vi "Construct_Remaining_Subtrack_101_2_Subtracks-1.vi"(0 "[IN] Still connected\ntracks in group":T2, 1 "[IN] Indexes for Jumps":i32[](array[numeric]), 5 "[IN] Clusters for Re\nconstructed Tracks":T1, 7 "[IN] Index of recon\nstructed tracks":i32, 11 "error IN":errorcluster, 12 "[IN] # column of re\nmaining elongation":i32, 13 "[IN] Indicies of Po\nints Inside Trks":i32[](array[numeric]), 14 "[IN] Indicies of all \nAffected Tracks \n(initial point = 0)":i32[](array[numeric])) -> (6 "[OUT] Clusters for Re\nconstructed Tracks":T1, 15 "error OUT":errorcluster)   [LabVIEW 2013]
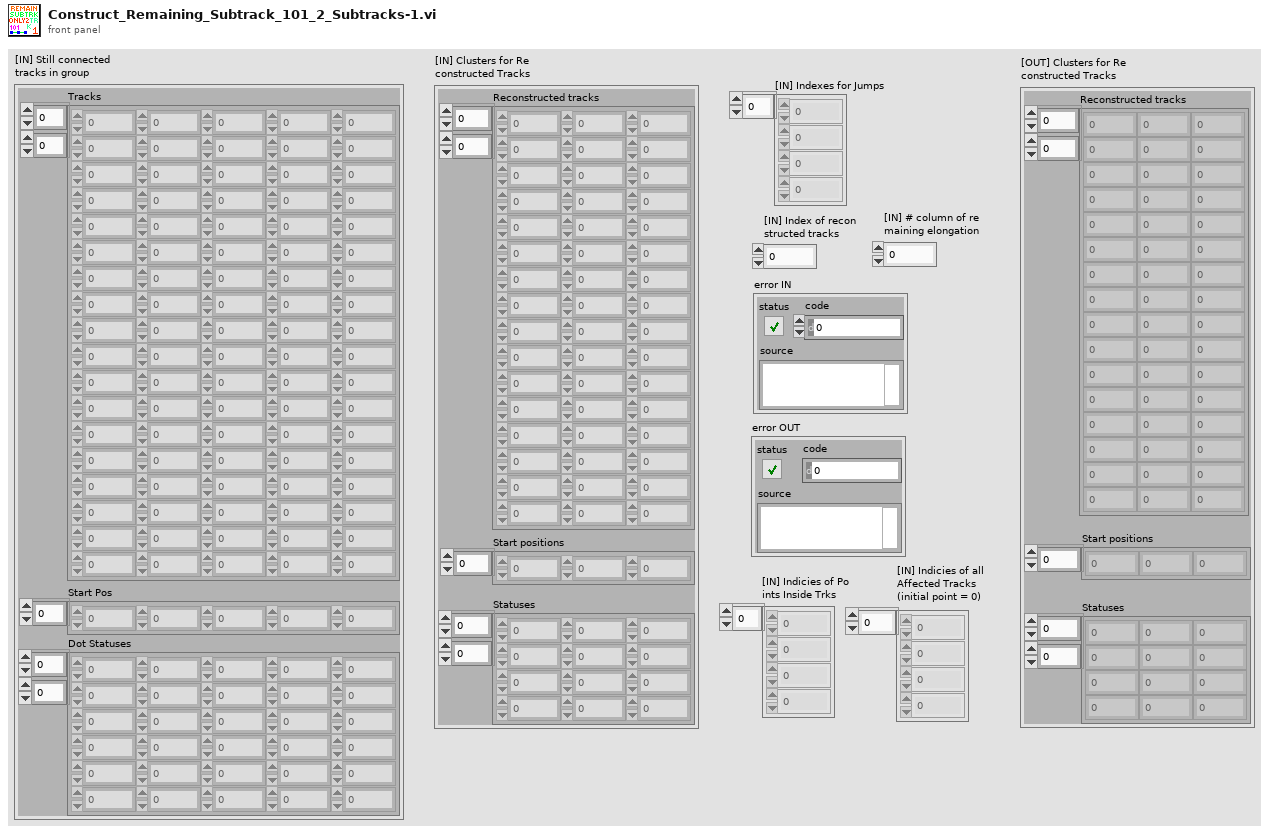
[diagram p1: front panel]
types:
  T1 = cluster{"Reconstructed tracks":dbl[][], "Start positions":i32[], "Statuses":i16[][]}
  T2 = cluster{"Tracks":dbl[][], "Start Pos":i32[], "Dot Statuses":i16[][]}
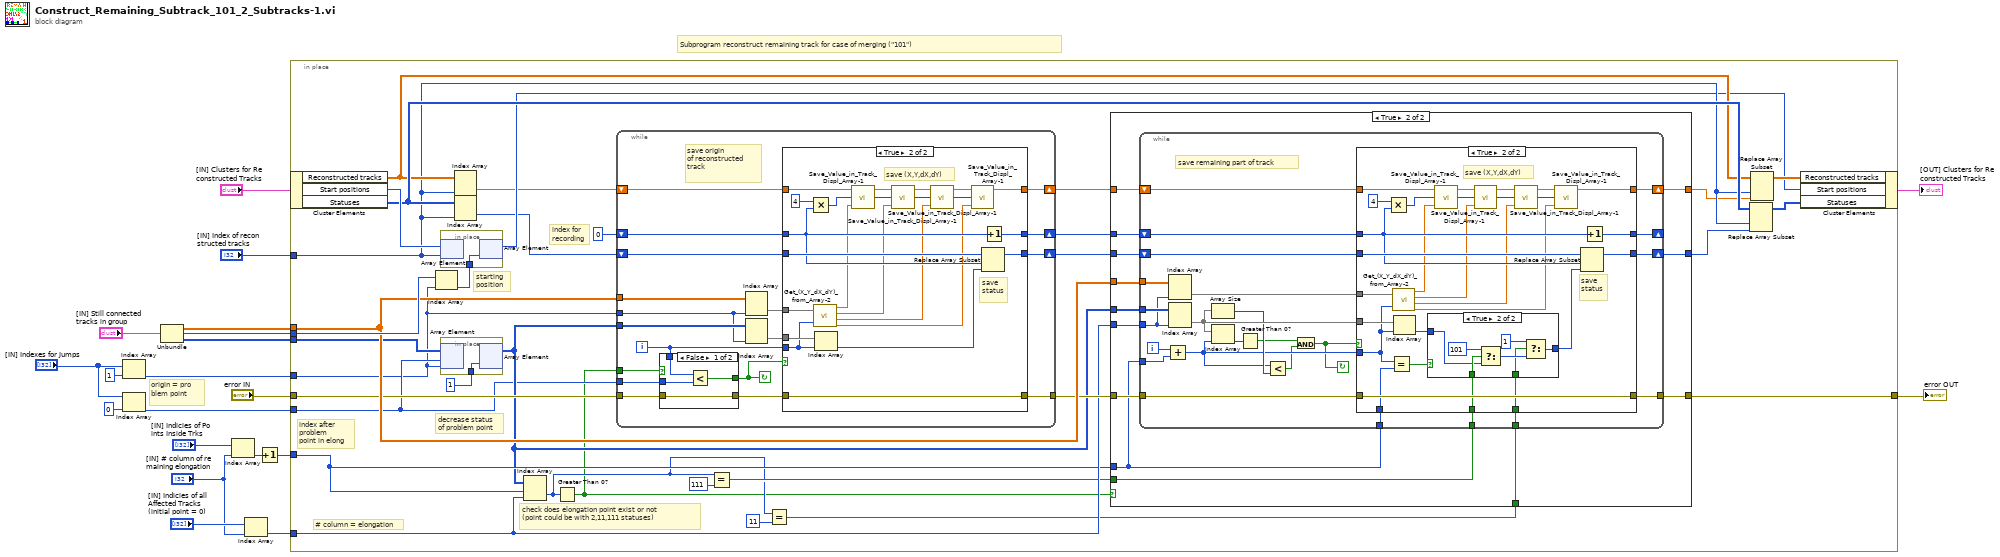
[diagram p0: block diagram]
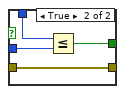
[diagram p5: hidden frame]
diagram:
  # "origin = pro\nblem point"
  # "Subprogram reconstruct remaining track for case of merging (\"101\")"
  n1 = Index Array(array="[IN] Indexes for Jumps", index=1) -> (element=w14:i32)
  n2 = Index Array(array="[IN] Indexes for Jumps", index=0) -> (element=w10:i32)
  n3 = Unbundle("[IN] Still connected\ntracks in group") -> ("Tracks"=w11:dbl[][], "Start Pos"=w12:i32[], "Dot Statuses"=w13:i16[][])
  n4 = Index Array(array="[IN] Indicies of Po\nints Inside Trks", index="[IN] # column of re\nmaining elongation") -> (element=w3:i32)
  n5 = Index Array(array="[IN] Indicies of all \nAffected Tracks \n(initial point = 0)", index="[IN] # column of re\nmaining elongation") -> (element=w5:i32)
  n6 = Increment(x=w3) -> (x+1=w2:i32)
  n7 = in-place {
    in-place-border: "[IN] Index of recon\nstructed tracks" -> [w49]
    in-place-border: w14 -> [w22]
    in-place-border: w13 -> [w29]
    in-place-border: w12 -> [w54]
    in-place-border: w11 -> [w53]
    in-place-border: w10 -> [w27]
    in-place-border: "error IN" -> [w48]
    in-place-border: w5 -> [w33]
    in-place-border: [w44] -> w7
    in-place-border: w2 -> [w32]
    # "decrease status\nof problem point"
    # "check does elongation point exist or not  \n(point could be with 2,11,111 statuses)"
    # "# column = elongation"
    # "index after\nproblem \npoint in elong"
    # "index for\nrecording"
    # "starting\nposition"
    n8 = in-place-cluster #1("[IN] Clusters for Re\nconstructed Tracks") -> ("Reconstructed tracks"=w50:dbl[][], "Start positions"=w52:i32[], "Statuses"=w51:i16[][])
    n9 = Index Array(array=w54, index=w22) -> (element=w43:i32)
    n10 = in-place {
      in-place-border: w43 -> [w189]
      n11 = in-place-array #2(w52, w49) -> ()  [unwired: 1 out]
      n12 = in-place-array #2(w189) -> (w46:i32[])  [unwired: 1 out]
    }
    n13 = in-place {
      in-place-border: i16 1 ("element") -> [w55]
      n14 = in-place-array #3(w29, w27, w22) -> ()  [unwired: 1 out]
      n15 = in-place-array #3(w55) -> (w28:i16[][])  [unwired: 2 out]
    }
    n16 = Index Array(array=w50, index (col)=w49) -> (element=w41:dbl[])  [unwired: 1 in]
    n17 = Index Array(array=w51, index (col)=w49) -> (element=w40:i16[])  [unwired: 1 in]
    n18 = Index Array(array=w28, index (row)=w32, index (col)=w33) -> (element=w24:i16)
    n19 = Greater Than 0?(x=w24) -> (x > 0?=w21:bool)
    n20 = while {
      tunnel: w27 -> [w139]
      tunnel: w53 -> [w153]
      tunnel: w28 -> [w152]
      tunnel: w22 -> [w151]
      shift-right: [w145] -> w39
      shift-left: w41 -> [w150]
      shift-right: [w143] -> w37
      shift-left: w40 -> [w147]
      shift-right: [w144] -> w38
      shift-left: 0 -> [w146]
      tunnel: w48 -> [w137]
      tunnel: [w142] -> w36
      tunnel: w21 -> [w141]
      i -> [w140]
      stop <- w138 continue-if-true
      # "save origin \nof reconstructed \ntrack"
      n21 = case shown="False" w141 {
        tunnel: w140 -> [w157 w161]
        tunnel: w139 -> [w156 w160]
        tunnel: [w155 w159] -> w138
        tunnel: w137 -> [w154 w158]
        tunnel: [w154 w158] -> w136
        frame False {
          n22 = Less?(x=w157, y=w156) -> (x < y?=w155:bool)
        }
        frame True {
          n23 = Less Or Equal?(x=w161, y=w160) -> (x <= y?=w159:bool)
        }
      }
      n24 = Index Array(array=w153, index (col)=w151) -> (element=w149:dbl[])  [unwired: 1 in]
      n25 = Index Array(array=w152, index (col)=w151) -> (element=w148:i16[])  [unwired: 1 in]
      n26 = case shown="True" w138 {
        tunnel: w150 -> [w165 w178]
        tunnel: w149 -> [_ w188]
        tunnel: w148 -> [_ w187]
        tunnel: w140 -> [_ w183]
        tunnel: w147 -> [w163 w185]
        tunnel: [w163 w182] -> w143
        tunnel: [w165 w167] -> w145
        tunnel: w146 -> [w164 w181]
        tunnel: [w164 w180] -> w144
        tunnel: w136 -> [w162 w179]
        tunnel: [w162 w179] -> w142
        frame False {
        }
        frame True {
          # "save (X,Y,dX,dY)"
          # "save\nstatus"
          n27 = Multiply(x=4, y=w181) -> (x*y=w176:i32)
          n28 = call "Get_(X_Y_dX_dY)_from_Array-2.vi"("(X,Y,dX,dY)"=w188, "Index of Displacement"=w183) -> ("X"=w177:dbl, "Y"=w173:dbl, "dX"=w171:dbl, "dY"=w168:dbl)
          n29 = Index Array(array=w187, index=w183) -> (element=w184:i16)
          n30 = call "Save_Value_in_Track_Displ_Array-1.vi"("[IN] Value"=w177, "[IN] Index"=w176, "[IN] Empty tracks\nfor points saving"=w178) -> ("[OUT] Index ++"=w174:i32, "[OUT Track with saved value"=w175:dbl[])  [unwired: 1 in]
          n31 = call "Save_Value_in_Track_Displ_Array-1.vi"("[IN] Value"=w173, "[IN] Index"=w174, "[IN] Empty tracks\nfor points saving"=w175) -> ("[OUT] Index ++"=w170:i32, "[OUT Track with saved value"=w172:dbl[])  [unwired: 1 in]
          n32 = call "Save_Value_in_Track_Displ_Array-1.vi"("[IN] Value"=w171, "[IN] Index"=w170, "[IN] Empty tracks\nfor points saving"=w172) -> ("[OUT] Index ++"=w166:i32, "[OUT Track with saved value"=w169:dbl[])  [unwired: 1 in]
          n33 = call "Save_Value_in_Track_Displ_Array-1.vi"("[IN] Value"=w168, "[IN] Index"=w166, "[IN] Empty tracks\nfor points saving"=w169) -> ("[OUT Track with saved value"=w167:dbl[])  [unwired: 1 in, 1 out]
          n34 = Replace Array Subset(array=w185, new element=w184, index=w181) -> (w182:i16[])
          n35 = Increment(x=w181) -> (x+1=w180:i32)
        }
      }
    }
    n36 = Equal?(x=w24, y=i16 111) -> (x = y?=w30:bool)
    n37 = Equal?(x=w24, y=i16 11) -> (x = y?=w23:bool)
    n38 = case shown="True" w21 {
      tunnel: w53 -> [_ w71]
      tunnel: [w56 w70] -> w44
      tunnel: w39 -> [w58 w69]
      tunnel: w38 -> [_ w68]
      tunnel: w37 -> [w57 w67]
      tunnel: w36 -> [w56 w66]
      tunnel: [w58 w65] -> w35
      tunnel: [w57 w64] -> w34
      tunnel: w28 -> [_ w63]
      tunnel: w33 -> [_ w62]
      tunnel: w32 -> [_ w60]
      tunnel: w30 -> [_ w61]
      tunnel: w23 -> [_ w59]
      frame False {
      }
      frame True {
        n39 = while {
          tunnel: w71 -> [w95]
          tunnel: w63 -> [w94]
          tunnel: w62 -> [w93]
          shift-right: [w88] -> w65
          shift-left: w69 -> [w92]
          shift-right: [w86] -> w64
          shift-left: w67 -> [w90]
          shift-right: [w87] -> _
          shift-left: w68 -> [w89]
          tunnel: w60 -> [w84]
          tunnel: w66 -> [w76]
          tunnel: [w75] -> w70
          tunnel: w60 -> [w74]
          tunnel: w61 -> [w73]
          tunnel: w59 -> [w72]
          i -> [w85]
          stop <- w77 continue-if-true
          # "save remaining part of track"
          n40 = Add(x=w85, y=w84) -> (x+y=w80:i32)
          n41 = Index Array(array=w95, index (col)=w93) -> (element=w91:dbl[])  [unwired: 1 in]
          n42 = Index Array(array=w94, index (col)=w93) -> (element=w83:i16[])  [unwired: 1 in]
          n43 = Array Size(array=w83) -> (size(s)=w81:i32)
          n44 = Index Array(array=w83, index=w80) -> (element=w82:i16)
          n45 = Greater Than 0?(x=w82) -> (x > 0?=w79:bool)
          n46 = Less?(x=w80, y=w81) -> (x < y?=w78:bool)
          n47 = And(x=w79, y=w78) -> (x .and. y?=w77:bool)
          n48 = case shown="True" w77 {
            tunnel: w92 -> [w99 w113]
            tunnel: w91 -> [_ w127]
            tunnel: w83 -> [_ w126]
            tunnel: w80 -> [_ w119]
            tunnel: w90 -> [w97 w124]
            tunnel: [w97 w123] -> w86
            tunnel: [w99 w101] -> w88
            tunnel: w89 -> [w98 w122]
            tunnel: [w98 w121] -> w87
            tunnel: w76 -> [w96 w120]
            tunnel: [w96 w120] -> w75
            tunnel: w74 -> [_ w118]
            tunnel: w73 -> [_ w114]
            tunnel: w72 -> [_ w100]
            frame False {
            }
            frame True {
              # "save (X,Y,dX,dY)"
              # "save\nstatus"
              n49 = Multiply(x=4, y=w122) -> (x*y=w112:i32)
              n50 = Equal?(x=w119, y=w118) -> (x = y?=w117:bool)
              n51 = call "Get_(X_Y_dX_dY)_from_Array-2.vi"("(X,Y,dX,dY)"=w127, "Index of Displacement"=w119) -> ("X"=w111:dbl, "Y"=w108:dbl, "dX"=w106:dbl, "dY"=w102:dbl)
              n52 = Index Array(array=w126, index=w119) -> (element=w116:i16)
              n53 = case shown="True" w117 {
                tunnel: w116 -> [w128 w133]
                tunnel: [w128 w131] -> w115
                tunnel: w114 -> [_ w135]
                tunnel: w100 -> [_ w129]
                frame False {
                }
                frame True {
                  n54 = Select(t=i16 101 ("element"), s=w135, f=w133) -> (s? t:f=w130:i16)
                  n55 = Select(t=i16 1 ("element"), s=w129, f=w130) -> (s? t:f=w131:i16)
                }
              }
              n56 = call "Save_Value_in_Track_Displ_Array-1.vi"("[IN] Value"=w111, "[IN] Index"=w112, "[IN] Empty tracks\nfor points saving"=w113) -> ("[OUT] Index ++"=w109:i32, "[OUT Track with saved value"=w110:dbl[])  [unwired: 1 in]
              n57 = call "Save_Value_in_Track_Displ_Array-1.vi"("[IN] Value"=w108, "[IN] Index"=w109, "[IN] Empty tracks\nfor points saving"=w110) -> ("[OUT] Index ++"=w105:i32, "[OUT Track with saved value"=w107:dbl[])  [unwired: 1 in]
              n58 = call "Save_Value_in_Track_Displ_Array-1.vi"("[IN] Value"=w106, "[IN] Index"=w105, "[IN] Empty tracks\nfor points saving"=w107) -> ("[OUT] Index ++"=w103:i32, "[OUT Track with saved value"=w104:dbl[])  [unwired: 1 in]
              n59 = call "Save_Value_in_Track_Displ_Array-1.vi"("[IN] Value"=w102, "[IN] Index"=w103, "[IN] Empty tracks\nfor points saving"=w104) -> ("[OUT Track with saved value"=w101:dbl[])  [unwired: 1 in, 1 out]
              n60 = Replace Array Subset(array=w124, new element=w115, index=w122) -> (w123:i16[])
              n61 = Increment(x=w122) -> (x+1=w121:i32)
            }
          }
        }
      }
    }
    n62 = Replace Array Subset(array=w51, new element=w34, index (col)=w49) -> (w45:i16[][])  [unwired: 1 in]
    n63 = Replace Array Subset(array=w50, new element=w35, index (col)=w49) -> (w47:dbl[][])  [unwired: 1 in]
    n64 = in-place-cluster #1("Reconstructed tracks"=w47, "Start positions"=w46, "Statuses"=w45) -> (→"[OUT] Clusters for Re\nconstructed Tracks":T1)
  }
  "error OUT" <- w7
